vi "Attacker.vi"(4 "balls":T1[](array[typedef]), 6 "geometry":T2, 10 "Robot":T3, 11 "command\nenum":T4) -> (2 "output cluster":T3)   [LabVIEW 2016]
uses:
  Core/AI Robot.ctl
  Command Enum.ctl
  Core/Field Size.ctl
  Core/AI Ball.ctl
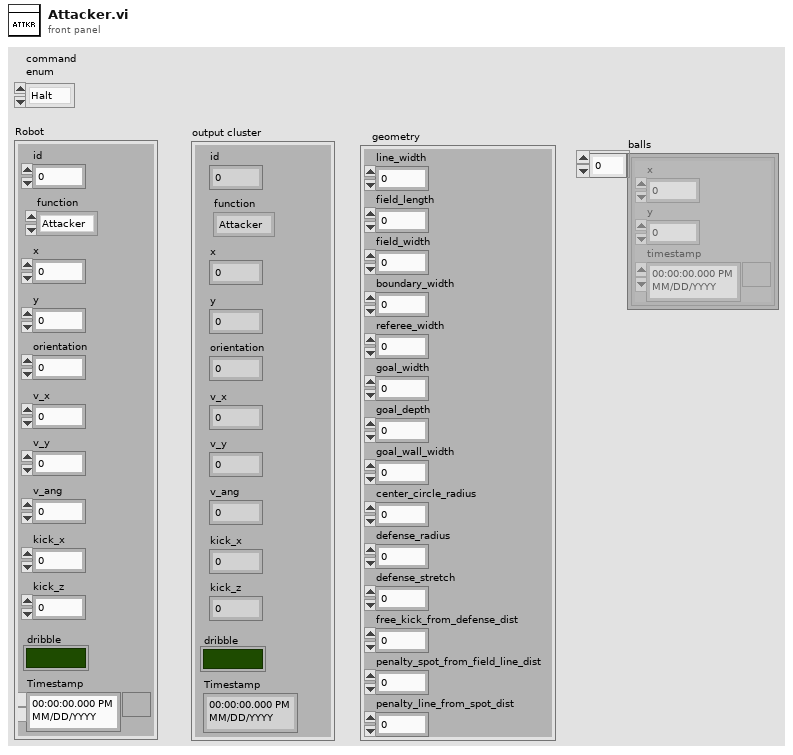
[diagram p1: front panel]
types:
  T1 = typedef "AI Ball.ctl" = cluster{"x":dbl, "y":dbl, "timestamp":timestamp}
  T2 = typedef "Field Size.ctl" = cluster{"line_width":u32, "field_length":u32, "field_width":u32, "boundary_width":u32, "referee_width":u32, "goal_width":u32, "goal_depth":u32, "goal_wall_width":u32, "center_circle_radius":u32, "defense_radius":u32, "defense_stretch":u32, "free_kick_from_defense_dist":u32, "penalty_spot_from_field_line_dist":u32, "penalty_line_from_spot_dist":u32}
  T3 = typedef "AI Robot.ctl" = cluster{"id":u32, "function":enum16{"Attacker", "Goalie", "Defender"}, "x":dbl, "y":dbl, "orientation":dbl, "v_x":dbl, "v_y":dbl, "v_ang":dbl, "kick_x":dbl, "kick_z":dbl, "dribble":bool, "Timestamp":timestamp}
  T4 = typedef "Command Enum.ctl" = enum16{"Halt", "Stop", "Force Start", "PKA Normal Start", "Prepare Kickoff Ally", "PKE Normal Start", "Prepare Kickoff Enemy", "Prepare Penalty Ally", "Prepare Penalty Enemy", "Direct Free Enemy", "Direct Free Ally", "Indirect Free Enemy", "Indirect Free Ally", "Timeout Enemy", "Timeout Ally", "Goal Enemy", "Goal Ally", "Ball Placement Enemy", "Ball Placement Ally", "None"}
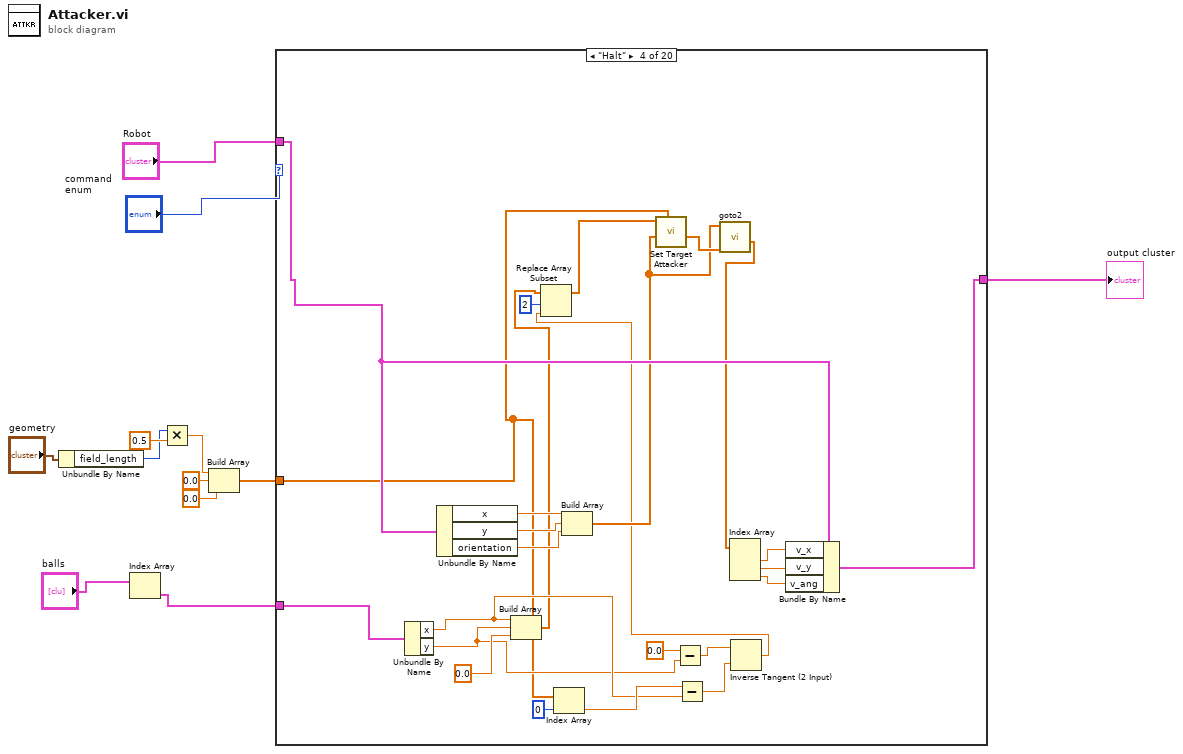
[diagram p0: block diagram]
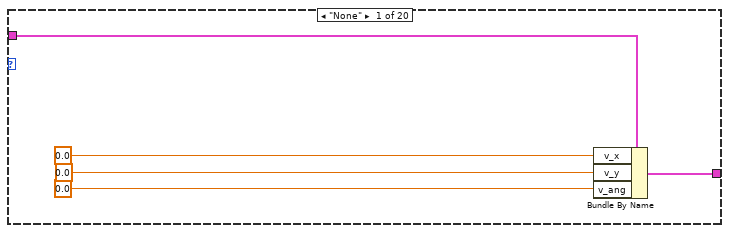
[diagram p2: hidden frame]
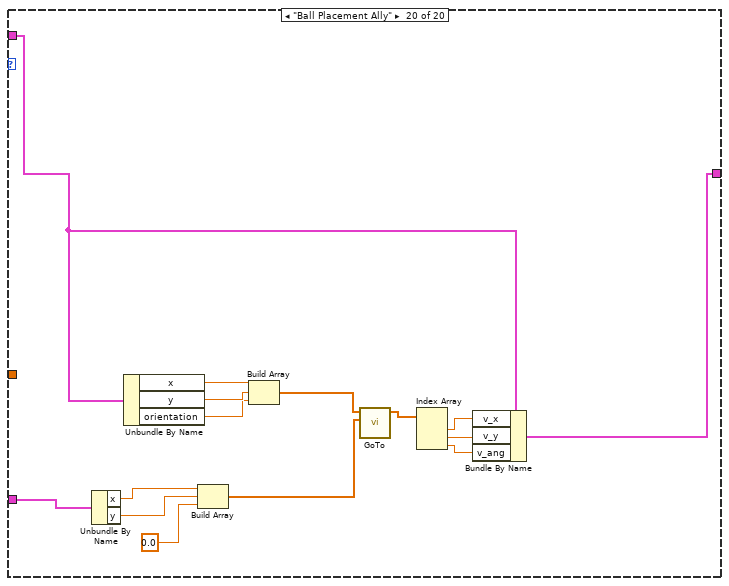
[diagram p20: hidden frame]
diagram:
  n1 = Unbundle By Name("geometry") -> ("field_length"=w5:u32)
  n2 = Index Array(array="balls") -> (element=w8:T1)  [unwired: 1 in]
  n3 = Multiply(x=w5, y=0.5) -> (x*y=w2:dbl)
  n4 = Build Array(w2, 0.0 ("element"), 0.0 ("element")) -> (w3:dbl[])
  n5 = case shown="\"Halt\"" "command\nenum" {
    tunnel: "Robot" -> [w17 w18 w19 w37 w45 w46 w47 w48 w49 w50 w51 w52 w53 w54 w55 w56 w57 w58 w59 w61]
    tunnel: [w13 w18 w19 w35 w45 w46 w47 w48 w49 w50 w51 w52 w53 w54 w55 w56 w57 w58 w59 w60] -> w10
    tunnel: w8 -> [_ _ _ w36 _ _ _ _ _ _ _ _ _ _ _ _ _ _ _ w70]
    tunnel: w3 -> [_ _ _ w20 _ _ _ _ _ _ _ _ _ _ _ _ _ _ _ _]
    frame "None" {
      n6 = Bundle By Name(cluster=w17, "v_x"=0.0, "v_y"=0.0, "v_ang"=0.0) -> (w13:T3)
    }
    frame Default {
    }
    frame "Stop" {
    }
    frame "Halt" {
      n7 = Unbundle By Name(w36) -> ("x"=w29:dbl, "y"=w27:dbl)
      n8 = Unbundle By Name(w37) -> ("x"=w38:dbl, "y"=w39:dbl, "orientation"=w40:dbl)
      n9 = Build Array(w29, w27, 0.0 ("element")) -> (w22:dbl[])
      n10 = Index Array(array=w20, index=0) -> (element=w30:dbl)
      n11 = Build Array(w38, w39, w40) -> (w32:dbl[])
      n12 = Subtract(x=0.0, y=w27) -> (x-y=w26:dbl)
      n13 = Subtract(x=w30, y=w29) -> (x-y=w25:dbl)
      n14 = Inverse Tangent (2 Input)(1:w25, 2:w26) -> (0:w24:dbl)
      n15 = Replace Array Subset(array=w22, new element=w24, index=2) -> (w21:dbl[])
      n16 = call "Set Target Attacker.vi"("GOAL"=w20, "Position"=w32, "Target"=w21) -> ("output"=w33:dbl[])  [unwired: 8 in]
      n17 = call "goto2.vi"("Target"=w33, "Pose"=w32) -> ("speed out"=w34:dbl[])  [unwired: 9 in]
      n18 = Index Array(array=w34) -> (element #1=w42:dbl, element #2=w43:dbl, element #3=w44:dbl)  [unwired: 3 in]
      n19 = Bundle By Name(cluster=w37, "v_x"=w42, "v_y"=w43, "v_ang"=w44) -> (w35:T3)
    }
    frame "PKA Normal Start" {
    }
    frame "Prepare Kickoff Ally" {
    }
    frame "PKE Normal Start" {
    }
    frame "Prepare Kickoff Enemy" {
    }
    frame "Prepare Penalty Ally" {
    }
    frame "Prepare Penalty Enemy" {
    }
    frame "Direct Free Enemy" {
    }
    frame "Direct Free Ally" {
    }
    frame "Indirect Free Enemy" {
    }
    frame "Indirect Free Ally" {
    }
    frame "Timeout Enemy" {
    }
    frame "Timeout Ally" {
    }
    frame "Goal Enemy" {
    }
    frame "Goal Ally" {
    }
    frame "Ball Placement Enemy" {
    }
    frame "Ball Placement Ally" {
      n20 = Unbundle By Name(w70) -> ("x"=w69:dbl, "y"=w68:dbl)
      n21 = Unbundle By Name(w61) -> ("x"=w74:dbl, "y"=w73:dbl, "orientation"=w72:dbl)
      n22 = Build Array(w69, w68, 0.0 ("element")) -> (w66:dbl[])
      n23 = Build Array(w74, w73, w72) -> (w71:dbl[])
      n24 = call "GoTo.vi"("Target"=w66, "Position"=w71) -> ("Output\nVelocity"=w65:dbl[])  [unwired: 9 in]
      n25 = Index Array(array=w65) -> (element #1=w64:dbl, element #2=w63:dbl, element #3=w62:dbl)  [unwired: 3 in]
      n26 = Bundle By Name(cluster=w61, "v_x"=w64, "v_y"=w63, "v_ang"=w62) -> (w60:T3)
    }
  }
  "output cluster" <- w10
